vi "Read Array refnum.vi"(8 "error in (no error)":errorcluster, 11 "Generic Prompt in":refnum<class "Generic Prompt.lvclass">) -> (0 "error out":errorcluster, 2 "Array refnum":refnum<vi>, 3 "Generic Prompt out":refnum<class "Generic Prompt.lvclass">)   [LabVIEW 2014, in "Generic Prompt.lvlib" / "Generic Prompt.lvclass"]
uses:
  Generic Prompt.lvclass
  Subpanel Insertion/Subpanel Inserter.lvclass
  Generic Prompt.lvclass/Generic Prompt.ctl
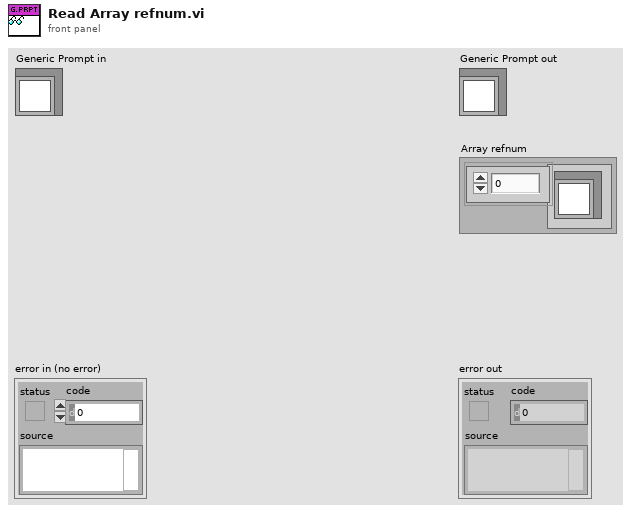
[diagram p1: front panel]
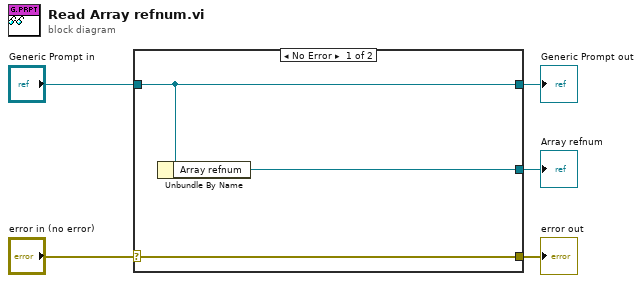
[diagram p0: block diagram]
diagram:
  n1 = case shown="No Error" "error in (no error)" {
    selector: "error in (no error)" -> [w8 w9]
    tunnel: [w8 w9] -> w4
    tunnel: [w7 w10] -> w2
    tunnel: "Generic Prompt in" -> [w7 w10]
    tunnel: [w6 _] -> w1
    frame No Error {
      n2 = Unbundle By Name(w7) -> ("Array refnum"=w6:refnum<vi>)
    }
    frame Error {
    }
  }
  "error out" <- w4
  "Generic Prompt out" <- w2
  "Array refnum" <- w1
